vi "GetString.vi"(7 "group":string, 8 "error in (no error)":errorcluster, 10 "param":string, 11 "_ConfigClass_INI_IN":refnum<class "_ConfigClass_INI.lvclass">) -> (0 "error out":errorcluster, 2 "string_out":string, 3 "_ConfigClass_INI_OUT":refnum<class "_ConfigClass_INI.lvclass">)   [LabVIEW 2019, in "_ConfigClass_INI.lvlib" / "_ConfigClass_INI.lvclass"]
uses:
  _ConfigClass_INI.lvclass
  _ConfigClass_INI.lvclass/_ConfigClass_INI.ctl
  <vilib>/Utility/config.llb/Read Key (String).vi
  <vilib>/Utility/config.llb/NI_LVConfig.lvlib
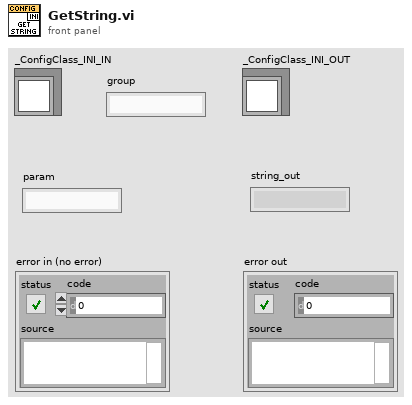
[diagram p1: front panel]
types:
  T1 = typedef "NI_LVConfig.lvlib/Config Data RefNum.ctl" = refnum<k1>
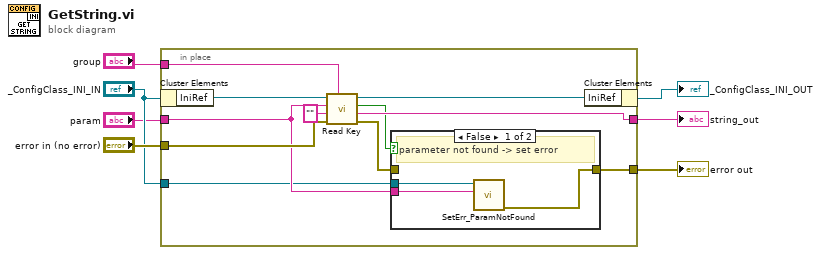
[diagram p0: block diagram]
diagram:
  n1 = in-place {
    in-place-border: "param" -> [w12]
    in-place-border: "error in (no error)" -> [w16]
    in-place-border: [w11] -> w5
    in-place-border: [w14] -> w4
    in-place-border: "_ConfigClass_INI_IN" -> [w9]
    in-place-border: "group" -> [w8]
    n2 = in-place-cluster #1("_ConfigClass_INI_IN") -> ("IniRef"=w18:T1)
    n3 = call-poly <vilib>:"Read Key.vi"("section"=w8, "error in (no error)"=w16, "default value"="", "key"=w12, "refnum"=w18) -> ("error out"=w13:errorcluster, "value"=w14:string, "found?"=w10:bool, "refnum out"=w17:T1)  [unwired: 3 in]
    n4 = case shown="False" w10 {
      tunnel: w13 -> [_ w22]
      tunnel: w12 -> [w20 _]
      tunnel: [w19 w22] -> w11
      tunnel: w9 -> [w21 _]
      frame False {
        # "parameter not found -> set error"
        n5 = call "SetErr_ParamNotFound.vi"("param"=w20, "_ConfigClass_INI.lvlib:_ConfigClass_INI_IN"=w21) -> ("error_OUT"=w19:errorcluster)  [unwired: 8 in, 1 out]
      }
      frame True {
        # "parameter found"
      }
    }
    n6 = in-place-cluster #1("IniRef"=w17) -> (→"_ConfigClass_INI_OUT":refnum<class "_ConfigClass_INI.lvclass">)
  }
  "error out" <- w5
  "string_out" <- w4
